vi "Error.vi"() -> ()   [LabVIEW 2018]
panel:
  in  "Boolean 10":bool
  in  "Boolean 9":bool
  in  "Boolean 8":bool
  in  "Boolean 7":bool
  in  "Boolean 6":bool
  in  "Boolean 5":bool
  in  "Table Control 2":string[][](table)=[["", "", "", "", "总压过压报警"], ["", "", "", "", "总压欠压报警"], ["", "", "", "", "绝缘电阻R+"], ["", "", "", "", "绝缘电阻R-"], ["", "", "", "", "单体电压上限"], ["", "", "", "", "单体电压下限"], ["", "", "", "", "单体压差告警"], ["", "", "", "", "瞬时温升过大告警"], ["", "", "", "", "单体温度上限"], ["", "", "", "", "单体温度下限"], ["", "", "", "", "单体SOC高"], ["", "", "", "", "单体SOC低"], ["", "", "", "", "放电电流告警"], ["", "", "", "", "充电电流告警"], ["", "", "", "", "温差过大告警"], ["", "", "", "", "高压盒温度过高告警"]]
  in  "Table Control":string[][](table)=[["", "", "", "", "总压过压报警"], ["", "", "", "", "总压欠压报警"], ["", "", "", "", "绝缘电阻R+"], ["", "", "", "", "绝缘电阻R-"], ["", "", "", "", "单体电压上限"], ["", "", "", "", "单体电压下限"], ["", "", "", "", "单体压差告警"], ["", "", "", "", "瞬时温升过大告警"], ["", "", "", "", "单体温度上限"], ["", "", "", "", "单体温度下限"], ["", "", "", "", "单体SOC高"], ["", "", "", "", "单体SOC低"], ["", "", "", "", "放电电流告警"], ["", "", "", "", "充电电流告警"], ["", "", "", "", "温差过大告警"], ["", "", "", "", "高压盒温度过高告警"]]
  in  "Boolean 4":bool
  in  "Boolean 3":bool
  in  "Boolean 2":bool
  in  "Boolean":bool
  # "BMS Monitor"
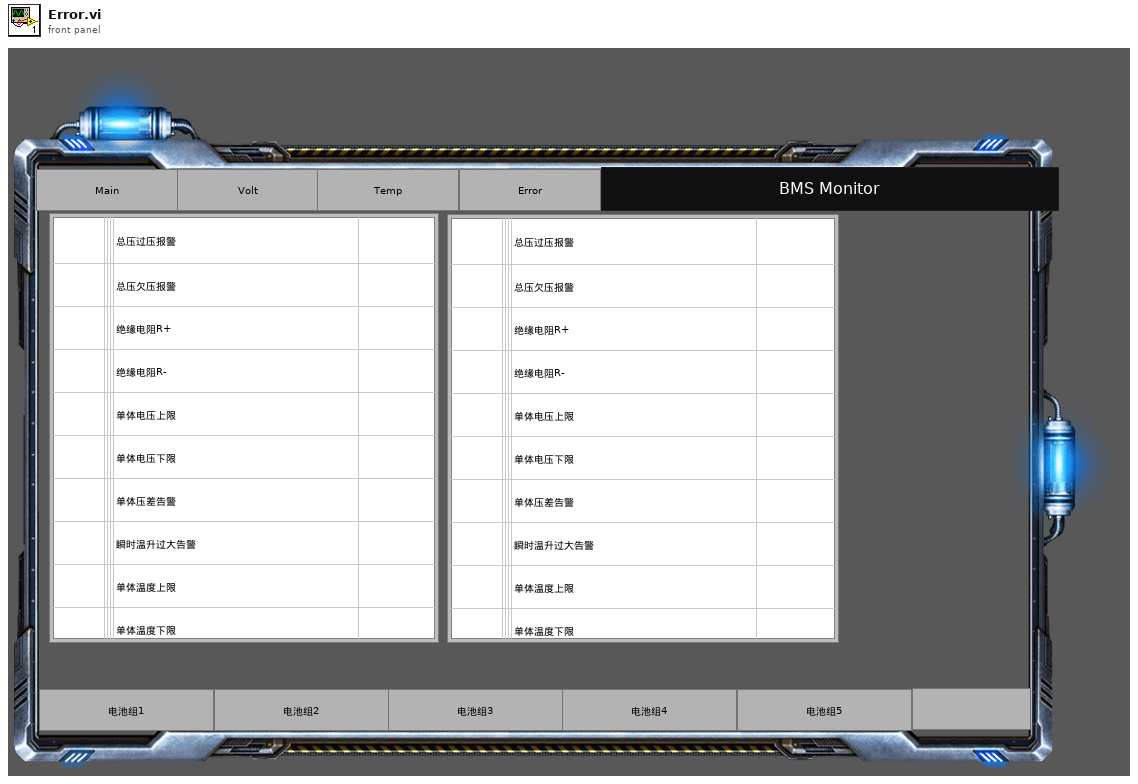
[diagram p1: front panel]
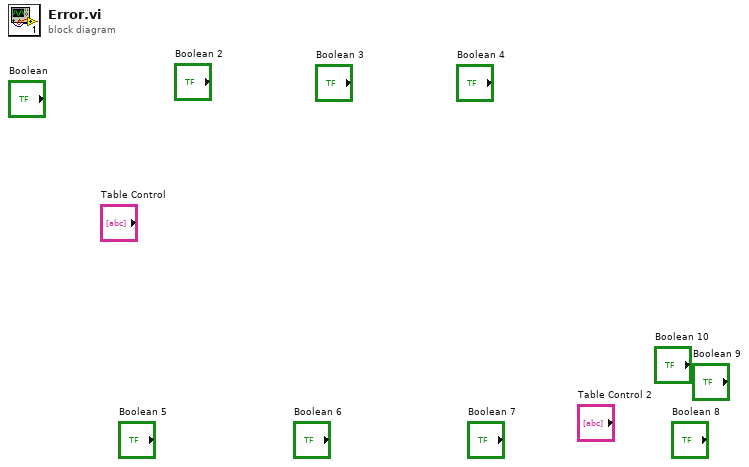
[diagram p0: block diagram]
diagram:
